vi "ForceCurveDecimated.vi"(6 "SaveArrayIn":dbl[][](array[numeric]), 7 "AcquiredChannels":i32[](listbox)=[0, 1, 2, 3], 8 "error in (no error)":errorcluster, 9 "InputParameters":T1, 10 "Data":fxp<+/-,18,1>[][](array[numeric]), 11 "GraphIn":cluster{dbl[], "Decimated Array":dbl[]}[](array[cluster])) -> (0 "error out":errorcluster, 1 "Fail":bool, 2 "PointsMax":i32, 3 "GraphOut":cluster{dbl[], "Decimated Array":dbl[]}[](array[cluster]), 4 "SaveArrayOut":dbl[][](array[numeric]))   [LabVIEW 2016]
uses:
  controls/Enum.ctl
  <vilib>/Analysis/2dsp.llb/Decimate (single shot, DBL).vi
  <vilib>/Utility/error.llb/Error Cluster From Error Code.vi
  <vilib>/rvi/errors/niLvFpgaAdjustHostInterfaceError.vi
  <vilib>/rvi/interface/nirviReadWriteControl/nirviReadWriteControl.xnode
  controls/FPGAVIreferenceTypeDef.ctl
  FPGA Bitfiles/qnmController797_usbRIO_controllerFPGAmu.lvbitx
  <vilib>/Analysis/NI_AALPro.lvlib
  NiFpgaLv.dll
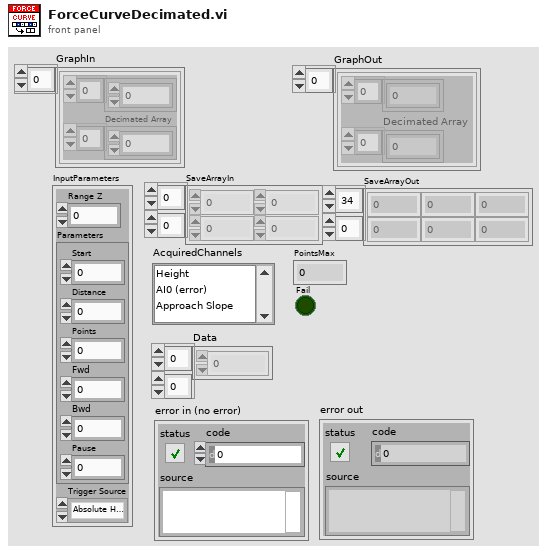
[diagram p1: front panel]
types:
  T1 = cluster{"Range Z":dbl, "Parameters":cluster{"Start":dbl, "Distance":dbl, "Points":dbl, "Fwd":dbl, "Bwd":dbl, "Pause":dbl}, "Trigger Source":enum16{"Absolute Height", "Process Variable", "External Source", "Relative Height"}}
  T2 = typedef "Enum.ctl" = enum16{"Init", "Read", "Write"}
  T3 = typedef "FPGAVIreferenceTypeDef.ctl" = refnum<k20>
  T4 = cluster{"Start":dbl, "Distance":dbl, "Points":dbl, "Fwd":dbl, "Bwd":dbl, "Pause":dbl}
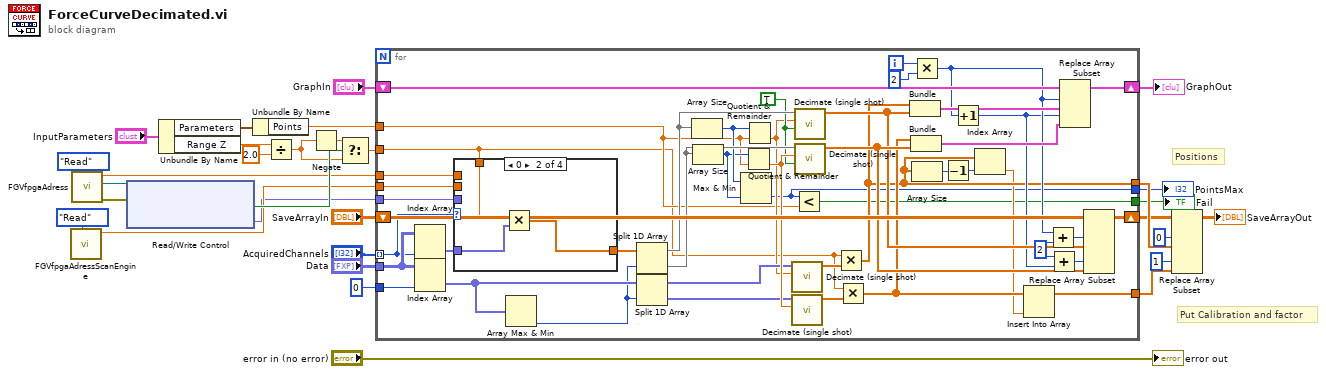
[diagram p0: block diagram]
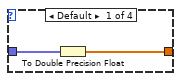
[diagram p2: hidden frame]
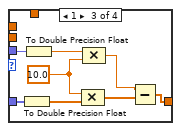
[diagram p3: hidden frame]
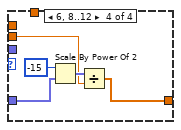
[diagram p4: hidden frame]
diagram:
  # "Put Calibration and factor"
  # "Positions"
  n1 = call "FGVfpgaAdressScanEngine.vi"("Enum"=Enum."Read") -> ("voltageRange(+/-)Out"=w5:dbl)  [unwired: 6 in, 4 out]
  n2 = call "FGVfpgaAdress.vi"("Enum"=Enum."Read") -> ("error out"=w12:errorcluster, "FPGA VI Reference Out"=w11:T3, "voltageRange(+/-)Out"=w6:dbl)  [unwired: 5 in, 3 out]
  n3 = xnode "Read/Write Control"("FPGA VI Reference In"=w11, "error in"=w12) -> ("aio.o.invertHeight"=w9:bool, "fb.p.params.setPoint"=w2:fxp<+/-,17,1>)  [unwired: 2 out]
  n4 = Unbundle By Name("InputParameters") -> ("Parameters"=w27:T4, "Range Z"=w16:dbl)
  n5 = Unbundle By Name(w27) -> ("Points"=w25:dbl)
  n6 = Divide(x=w16, y=2.0) -> (x/y=w1:dbl)
  n7 = Negate(x=w1) -> (-x=w8:dbl)
  n8 = Select(t=w8, s=w9, f=w1) -> (s? t:f=w10:dbl)
  n9 = for {
    tunnel: "Data" -> [w73]
    tunnel: "AcquiredChannels" -> [w36] mode=indexing
    shift-right: [w72] -> w30
    shift-left: "GraphIn" -> [w67]
    shift-right: [w71] -> w23
    shift-left: "SaveArrayIn" -> [w77]
    tunnel: w25 -> [w41]
    tunnel: w10 -> [w32]
    tunnel: [w46] -> w24
    tunnel: 0 ("disabled index (col)") -> [w62]
    tunnel: [w48] -> w14
    tunnel: w6 -> [w35]
    tunnel: w5 -> [w34]
    tunnel: [w39] -> w4
    tunnel: [w40] -> w3
    tunnel: w2 -> [w33]
    i -> [w66]
    w52 = 2 ("x")
    w70 = TRUE ("averaging")
    n10 = Index Array(array=w73, index (col)=w36) -> (element=w38:fxp<+/-,18,1>[])  [unwired: 1 in]
    n11 = Index Array(array=w73, index (col)=w62) -> (element=w61:fxp<+/-,18,1>[])  [unwired: 1 in]
    n12 = case shown="0" w36 {
      tunnel: w38 -> [w79 w81 w89 w92]
      tunnel: w35 -> [_ _ _ _]
      tunnel: w34 -> [_ _ _ w91]
      tunnel: [w78 w82 w83 w93] -> w37
      tunnel: w33 -> [_ _ w90 _]
      tunnel: w32 -> [_ w80 _ _]
      frame Default {
        n13 = To Double Precision Float(number=w79) -> (double precision float=w78:dbl[])
      }
      frame 0 {
        n14 = Multiply(x=w80, y=w81) -> (x*y=w82:dbl[])
      }
      frame 1 {
        w87 = 10.0
        n15 = To Double Precision Float(number=w89) -> (double precision float=w88:dbl[])
        n16 = To Double Precision Float(number=w90) -> (double precision float=w86:dbl)
        n17 = Compound Arithmetic op=MULTIPLY(w87, w88) -> (w85:dbl[])
        n18 = Compound Arithmetic op=MULTIPLY(w86, w87) -> (w84:dbl)
        n19 = Subtract(x=w84, y=w85) -> (x-y=w83:dbl[])
      }
      frame 6, 8..12 {
        n20 = Scale By Power Of 2(n=i16 -15, x=w92) -> (x*2^n=w94:fxp<+/-,18,1>[])
        n21 = Divide(x=w94, y=w91) -> (x/y=w93:dbl[])
      }
    }
    n22 = Array Max & Min(array=w61) -> (min index (indices)=w60:i32)  [unwired: 3 out]
    n23 = Split 1D Array(array=w37, index=w60) -> (first subarray=w76:dbl[], second subarray=w75:dbl[])
    n24 = Split 1D Array(array=w61, index=w60) -> (first subarray=w59:fxp<+/-,18,1>[], second subarray=w51:fxp<+/-,18,1>[])
    n25 = Array Size(array=w76) -> (size(s)=w43:i32)
    n26 = Array Size(array=w75) -> (size(s)=w42:i32)
    n27 = Max & Min(x=w43, y=w42) -> (min(x,y)=w39:i32)  [unwired: 1 out]
    n28 = Quotient & Remainder(x=w42, y=w41) -> (floor(x/y)=w74:dbl)  [unwired: 1 out]
    n29 = Quotient & Remainder(x=w43, y=w41) -> (floor(x/y)=w56:dbl)  [unwired: 1 out]
    n30 = call-poly <vilib>:"Decimate (single shot).vi"("decimating factor"=w56, "X"=w59) -> ("Decimated Array"=w58:dbl[])  [unwired: 8 in, 1 out]
    n31 = call-poly <vilib>:"Decimate (single shot).vi"("decimating factor"=w74, "X"=w51) -> ("Decimated Array"=w57:dbl[])  [unwired: 8 in, 1 out]
    n32 = Less?(x=w39, y=w41) -> (x < y?=w40:bool)
    n33 = call-poly <vilib>:"Decimate (single shot).vi"("averaging"=w70, "decimating factor"=w56, "X"=w76) -> ("Decimated Array"=w54:dbl[])  [unwired: 7 in, 1 out]
    n34 = call-poly <vilib>:"Decimate (single shot).vi"("averaging"=w70, "decimating factor"=w74, "X"=w75) -> ("Decimated Array"=w55:dbl[])  [unwired: 7 in, 1 out]
    n35 = Multiply(x=w32, y=w58) -> (x*y=w46:dbl[])
    n36 = Multiply(x=w32, y=w57) -> (x*y=w49:dbl[])
    n37 = Bundle(w46, "Decimated Array"=w54) -> (w69:cluster{dbl[], "Decimated Array":dbl[]})  [unwired: 1 in]
    n38 = Bundle(w49, "Decimated Array"=w55) -> (w68:cluster{dbl[], "Decimated Array":dbl[]})  [unwired: 1 in]
    n39 = Multiply(x=w66, y=2) -> (x*y=w53:i32)
    n40 = Array Size(array=w46) -> (size(s)=w47:i32)
    n41 = Decrement(x=w47) -> (x-1=w45:i32)
    n42 = Increment(x=w53) -> (x+1=w50:i32)
    n43 = Index Array(array=w46, index=w45) -> (element=w44:dbl)
    n44 = Insert Into Array(array=w49, new element=w44) -> (w48:dbl[])  [unwired: 1 in]
    n45 = Add(x=w53, y=w52) -> (x+y=w64:i32)
    n46 = Add(x=w52, y=w50) -> (x+y=w63:i32)
    n47 = Replace Array Subset(array=w67, new element #1=w69, index #1=w53, new element #2=w68, index #2=w50) -> (w72:cluster{dbl[], "Decimated Array":dbl[]}[])
    n48 = Replace Array Subset(array=w77, new element #1=w54, index (col) #1=w64, new element #2=w55, index (col) #2=w63) -> (w71:dbl[][])  [unwired: 2 in]
  }
  "GraphOut" <- w30
  "PointsMax" <- w4
  "Fail" <- w3
  n49 = Replace Array Subset(array=w23, new element #1=w24, index (col) #1=0 ("disabled index (col)"), new element #2=w14, index (col) #2=1 ("index (col)")) -> (→"SaveArrayOut":dbl[][])  [unwired: 2 in]
  "error out" <- "error in (no error)"
